vi "Configure Counter Unit.vi"(8 "error in (no error)":errorcluster, 9 "Counter Unit (-1:Select a Unit)":i32(ring)=-1 items=["Select a Unit"=-1, "l"=10, "mm3"=11, "ml"=12, "cm3"=13, "ul"=14, "m3"=15, "g"=20, "mg"=21, "ug"=22, "kg"=23, "ln"=30, "mm3n"=31, "mln"=32, "cm3n"=33, "uln"=34, "dm3n"=35, "m3n"=36, "uls"=37, "mm3s"=38, "mls"=39, "cm3s"=40, "ls"=41, "dm3s"=42, "m3s"=43], 10 "Node (3)":u8=3 min=3 max=128 step=1, 11 "VISA resource name":refnum<visa-resource-name>) -> (0 "error out":errorcluster, 3 "VISA resource name out":refnum<visa-resource-name>)   [LabVIEW 2019, in "Bronkhorst FLOW-BUS.lvlib"]
doc: "Configures the unit that the counter counts."
uses:
  Bronkhorst FLOW-BUS.lvlib
  Private/FLOW-BUS RW.ctl
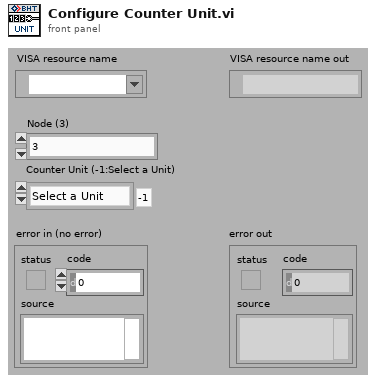
[diagram p1: front panel]
types:
  T1 = typedef "Bronkhorst FLOW-BUS.lvlib/FLOW-BUS RW.ctl" = cluster{"Node Address (3)":u8, "Communication Command":enum16{"Status message", "Send parameter with destination address and 00 response", "Send parameter with destination address", "Request parameter"}, "Process (0)":u16, "Parameter (0)":u16, "Data Type (0: Character)":enum16{"Character", "Integer", "Float or Long", "String"}, "Data for Char or Int (0)":u32, "Data for Float or Long (0)":sgl, "Data for String":string, "Length of Requested String (0)":u8}
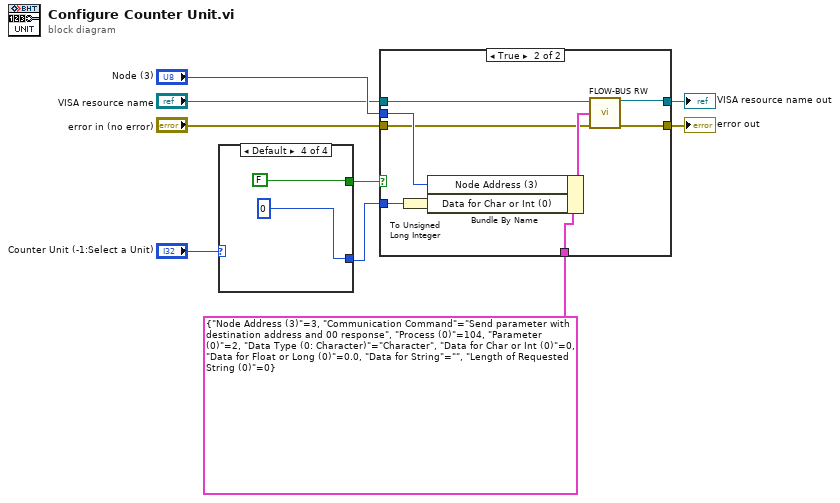
[diagram p0: block diagram]
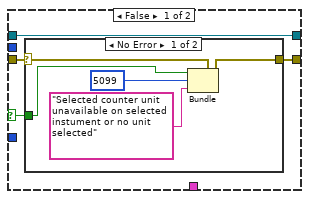
[diagram p2: hidden frame]
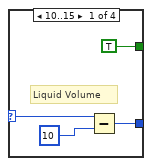
[diagram p4: hidden frame]
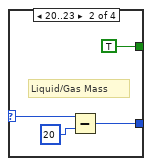
[diagram p5: hidden frame]
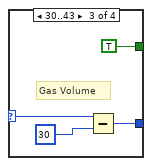
[diagram p6: hidden frame]
diagram:
  n1 = case shown="Default" "Counter Unit (-1:Select a Unit)" {
    selector: "Counter Unit (-1:Select a Unit)" -> [w11 w16 w20 _]
    tunnel: [w12 w15 w19 0] -> w4
    tunnel: [TRUE TRUE TRUE FALSE] -> w8
    frame 10..15 {
      # "Liquid Volume"
      n2 = Subtract(x=w11, y=10) -> (x-y=w12:i32)
    }
    frame 20..23 {
      # "Liquid/Gas Mass"
      n3 = Subtract(x=w16, y=20) -> (x-y=w15:i32)
    }
    frame 30..43 {
      # "Gas Volume"
      n4 = Subtract(x=w20, y=30) -> (x-y=w19:i32)
    }
    frame Default {
    }
  }
  n5 = case shown="True" w8 {
    selector: w8 -> [w24 _]
    tunnel: "VISA resource name" -> [w27 w36]
    tunnel: "error in (no error)" -> [w26 w37]
    tunnel: "Node (3)" -> [_ w39]
    tunnel: [w27 w35] -> w7
    tunnel: [w25 w34] -> w6
    tunnel: w4 -> [_ w40]
    tunnel: T1 {"Node Address (3)"=3, "Communication Command"=enum."Send parameter with destination address and 00 response", "Process (0)"=104, "Parameter (0)"=2, "Data Type (0: Character)"=enum."Character", "Data for Char or Int (0)"=0, "Data for Float or Long (0)"=0.0, "Data for String"="", "Length of Requested String (0)"=0} ("FLOW-BUS Command Settings") -> [_ w41]
    frame False {
      n6 = case shown="No Error" w26 {
        selector: w26 -> [w30 w33]
        tunnel: [w29 w33] -> w25
        tunnel: w24 -> [w28 _]
        frame No Error {
          n7 = Bundle(cluster=w30, "status"=w28, "code"=5099, "source"="Selected counter unit unavailable on selected instument or no unit selected") -> (w29:errorcluster)
        }
        frame Error {
        }
      }
    }
    frame True {
      n8 = To Unsigned Long Integer(number=w40) -> (unsigned 32bit integer=w42:u32)
      n9 = Bundle By Name(cluster=w41, "Node Address (3)"=w39, "Data for Char or Int (0)"=w42) -> (w38:T1)
      n10 = call "FLOW-BUS RW.vi"("VISA resource name"=w36, "FLOW-BUS Command Settings"=w38, "error in (no error)"=w37) -> ("VISA resource name out"=w35:refnum<visa-resource-name>, "error out"=w34:errorcluster)  [unwired: 8 in, 3 out]
    }
  }
  "error out" <- w6
  "VISA resource name out" <- w7
